vi "Charge and Discharge.vi"(8 "TDMS File Path In":string, 9 "Voltage":dbl=1.5, 10 "Initial Capacity  (mAh)":dbl=2350.0, 11 "Cycle":i32) -> (0 "TDMS File Path":string, 1 "Passed":bool, 2 "Energy (Wh)":dbl, 3 "Capacity (mAh)":dbl)   [LabVIEW 2019]
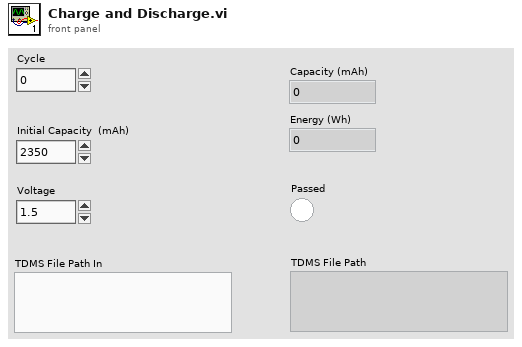
[diagram p1: front panel]
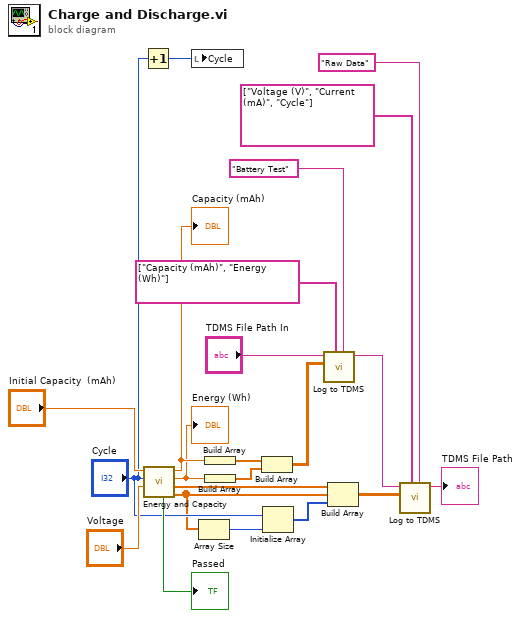
[diagram p0: block diagram]
diagram:
  n1 = Increment(x="Cycle") -> (x+1=w20:i32)
  n2 = call "Energy and Capacity.vi"("Voltage"="Voltage", "Cycle"="Cycle", "Initial Capacity  (mAh) in"="Initial Capacity  (mAh)") -> ("Current (mA)"=w1:dbl[], "Voltage (V)"=w9:dbl[], "Energy (Wh)"=w18:dbl, "Capacity  (mAh)"=w19:dbl, "Pass"=→"Passed":bool)  [unwired: 4 in]
  "Energy (Wh)" <- w18
  "Capacity (mAh)" <- w19
  n3 = local write "Cycle"(w20) -> ()
  n4 = Array Size(array=w1) -> (size(s)=w2:i32)
  n5 = Build Array(w19) -> (w17:dbl[])
  n6 = Build Array(w18) -> (w16:dbl[])
  n7 = Build Array(w17, w16) -> (w12:dbl[][])
  n8 = Initialize Array("Cycle", w2) -> (w3:i32[])
  n9 = call "Log to TDMS.vi"("group name in (Untitled)"="Battery Test", "channel name(s) in (Untitled)"=string[] ["Capacity (mAh)", "Energy (Wh)"], "Array"=w12, "TDMS File Path In"="TDMS File Path In") -> ("String"=w10:string)  [unwired: 7 in]
  n10 = Build Array(w9, w1, w3) -> (w8:dbl[][])
  n11 = call "Log to TDMS.vi"("group name in (Untitled)"="Raw Data", "channel name(s) in (Untitled)"=string[] ["Voltage (V)", "Current (mA)", "Cycle"], "Array"=w8, "TDMS File Path In"=w10) -> ("String"=→"TDMS File Path":string)  [unwired: 7 in]
